vi "Localize This VI.vi"   [LabVIEW 2019]
types:
  T1 = enum32{"invalid OS target", "Mac OS", "Windows 3.1", "Windows 95/NT", "Solaris 1", "Solaris 2", "HP-UX", "PowerMAX", "Linux", "Irix", "Rhapsody", "BeOS", "AIX", "OSF1", "VxWorks", "PharLap", "Carbon", "RTX", "Windows x64", "Linux x64", "Mac OS X x64"}
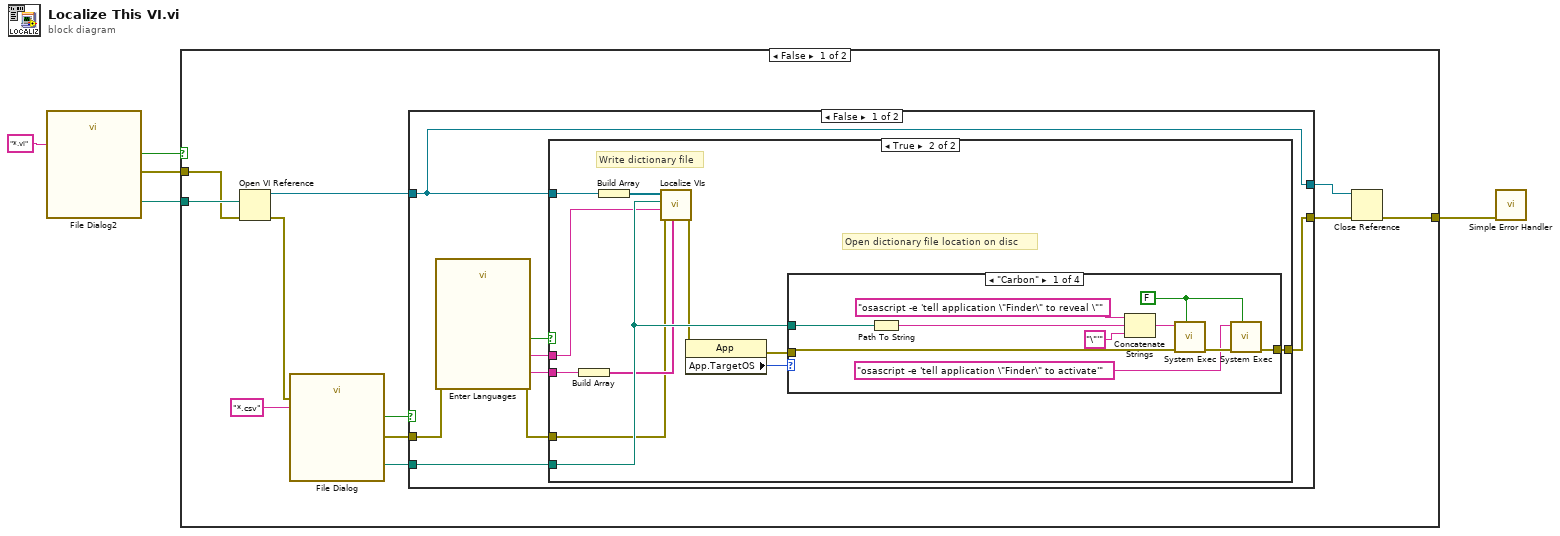
[diagram p0: block diagram]
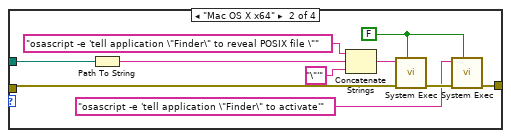
[diagram p3: hidden frame]
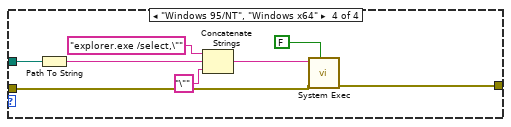
[diagram p5: hidden frame]
diagram:
  n1 = call "File Dialog2"("pattern (all files)"="*.vi" ("pattern label")) -> ("selected path"=w3:path, "cancelled"=w1:bool, "error out"=w2:errorcluster)  [unwired: 11 in, 1 out]
  n2 = case shown="False" w1 {
    tunnel: [w8 w68] -> w5
    tunnel: w3 -> [w7 _]
    tunnel: w2 -> [w6 w68]
    frame False {
      n3 = Open VI Reference(vi path=w7, error in (no error)=w6) -> (vi reference=w15:refnum<vi>, error out=w16:errorcluster)  [unwired: 4 in]
      n4 = call "File Dialog"("error in"=w16, "pattern (all files)"="*.csv" ("pattern label")) -> ("selected path"=w14:path, "cancelled"=w12:bool, "error out"=w13:errorcluster)  [unwired: 10 in, 1 out]
      n5 = case shown="False" w12 {
        tunnel: w15 -> [w24 w67]
        tunnel: w14 -> [w23 _]
        tunnel: w13 -> [w19 w66]
        tunnel: [w24 w67] -> w11
        tunnel: [w22 w66] -> w10
        frame False {
          n6 = call "Enter Languages"("error in (no error)"=w19) -> ("Additional Language"=w20:string, "Current Language"=w21:string, "OK"=w17:bool, "error out"=w18:errorcluster)  [unwired: 15 in]
          n7 = case shown="True" w17 {
            tunnel: w24 -> [_ w35]
            tunnel: w23 -> [_ w33]
            tunnel: [w25 w30] -> w22
            tunnel: w21 -> [_ w29]
            tunnel: w20 -> [_ w28]
            tunnel: w18 -> [w25 w26]
            frame False {
            }
            frame True {
              # "Open dictionary file location on disc"
              # "Write dictionary file"
              n8 = Build Array(w28) -> (w27:string[])
              n9 = Build Array(w35) -> (w36:refnum<vi>[])
              n10 = call "Localize VIs.vi"("Additional Languages [English]"=w27, "error in (no error)"=w26, "Current VI Language (English)"=w29, "Dictionary Path"=w33, "VIs in"=w36) -> ("error out"=w32:errorcluster)  [unwired: 6 in]
              n11 = property class="App"(error in=w32) -> (error out=w31:errorcluster, "App.TargetOS"=w34:T1)  [unwired: 1 in, 1 out]
              n12 = case shown="\"Carbon\"" w34 {
                tunnel: w33 -> [w39 w51 _ w61]
                tunnel: w31 -> [w37 w47 w57 w59]
                tunnel: [w38 w48 w57 w58] -> w30
                frame "Carbon" {
                  w42 = FALSE ("wait until completion? (T)")
                  n13 = Path To String(path=w39) -> (string=w40:string)
                  n14 = Concatenate Strings("osascript -e 'tell application \"Finder\" to reveal \"" ("string"), w40, "\"'" ("string")) -> (w44:string)
                  n15 = call <vilib>:"System Exec.vi"("wait until completion? (T)"=w42, "error in (no error)"=w37, "command line"=w44) -> ("error out"=w43:errorcluster)  [unwired: 5 in, 3 out]
                  n16 = call <vilib>:"System Exec.vi"("wait until completion? (T)"=w42, "error in (no error)"=w43, "command line"="osascript -e 'tell application \"Finder\" to activate'" ("string")) -> ("error out"=w38:errorcluster)  [unwired: 5 in, 3 out]
                }
                frame "Mac OS X x64" {
                  w53 = FALSE ("wait until completion? (T)")
                  n17 = Path To String(path=w51) -> (string=w50:string)
                  n18 = Concatenate Strings("osascript -e 'tell application \"Finder\" to reveal POSIX file \"" ("string"), w50, "\"'" ("string")) -> (w55:string)
                  n19 = call <vilib>:"System Exec.vi"("wait until completion? (T)"=w53, "error in (no error)"=w47, "command line"=w55) -> ("error out"=w54:errorcluster)  [unwired: 5 in, 3 out]
                  n20 = call <vilib>:"System Exec.vi"("wait until completion? (T)"=w53, "error in (no error)"=w54, "command line"="osascript -e 'tell application \"Finder\" to activate'" ("string")) -> ("error out"=w48:errorcluster)  [unwired: 5 in, 3 out]
                }
                frame Default {
                }
                frame "Windows 95/NT", "Windows x64" {
                  n21 = Path To String(path=w61) -> (string=w60:string)
                  n22 = Concatenate Strings("explorer.exe /select,\"" ("string"), w60, "\"" ("string")) -> (w63:string)
                  n23 = call <vilib>:"System Exec.vi"("wait until completion? (T)"=FALSE, "error in (no error)"=w59, "command line"=w63) -> ("error out"=w58:errorcluster)  [unwired: 5 in, 3 out]
                }
              }
            }
          }
        }
        frame True {
        }
      }
      n24 = Close Reference(reference=w11, error in (no error)=w10) -> (error out=w8:errorcluster)
    }
    frame True {
    }
  }
  n25 = call <vilib>:"Simple Error Handler.vi"("error in (no error)"=w5) -> ()  [unwired: 4 in, 5 out]
